vi "Ping.vi"(8 "error in (no error)":errorcluster, 10 "IP":string) -> (0 "error out":errorcluster, 2 "Active":bool)   [LabVIEW 2022 SP3, in "TouchControl.lvlib"]
uses:
  TouchControl.lvlib
panel:
  out "standard output":string
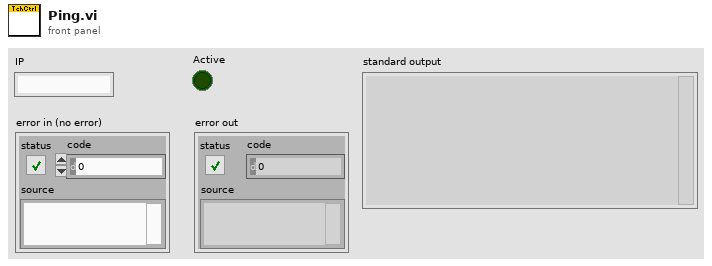
[diagram p1: front panel]
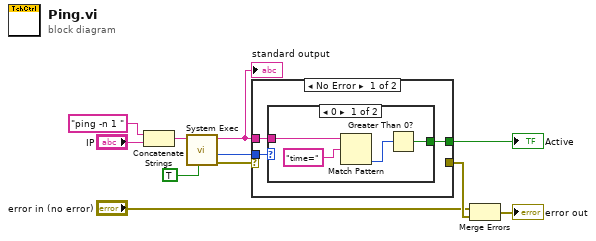
[diagram p0: block diagram]
diagram:
  n1 = Concatenate Strings("ping -n 1 " ("format string"), "IP") -> (w9:string)
  n2 = call <vilib>:"System Exec.vi"("run minimized? (F)"=TRUE, "command line"=w9) -> ("error out"=w5:errorcluster, "return code"=w8:i32, "standard output"=w7:string)  [unwired: 6 in, 1 out]
  "standard output" <- w7
  n3 = case shown="No Error" w5 {
    selector: w5 -> [_ w19]
    tunnel: w8 -> [w14 _]
    tunnel: w7 -> [w13 _]
    tunnel: [w12 _] -> w6
    tunnel: [_ w19] -> w4
    frame No Error {
      n4 = case shown="0" w14 {
        tunnel: w13 -> [w18 _]
        tunnel: [w15 _] -> w12
        frame 0 {
          n5 = Match Pattern(string=w18, regular expression="time=") -> (offset past match=w16:i32)  [unwired: 1 in, 3 out]
          n6 = Greater Than 0?(x=w16) -> (x > 0?=w15:bool)
        }
        frame Default {
        }
      }
    }
    frame Error {
    }
  }
  "Active" <- w6
  n7 = Merge Errors("error in (no error)", w4) -> (→"error out":errorcluster)
